vi "zadanie 3.vi"() -> ()   [LabVIEW 2013]
panel:
  out "Meter":dbl(knob) scale=0.0..1.0
  in  "Управление":bool
  out "Напряжение":dbl[](graph)
  out "Тестовый массив":dbl[](array[numeric])
  in  "С":dbl
  out "Заряд стикающий с конденсатора":dbl[](graph)
  out "Сила тока на нагрузке":dbl[](graph)
  out "t":dbl
  out "I":dbl
  out "Q":dbl
  in  "R":dbl
  in  "ЭДС":dbl
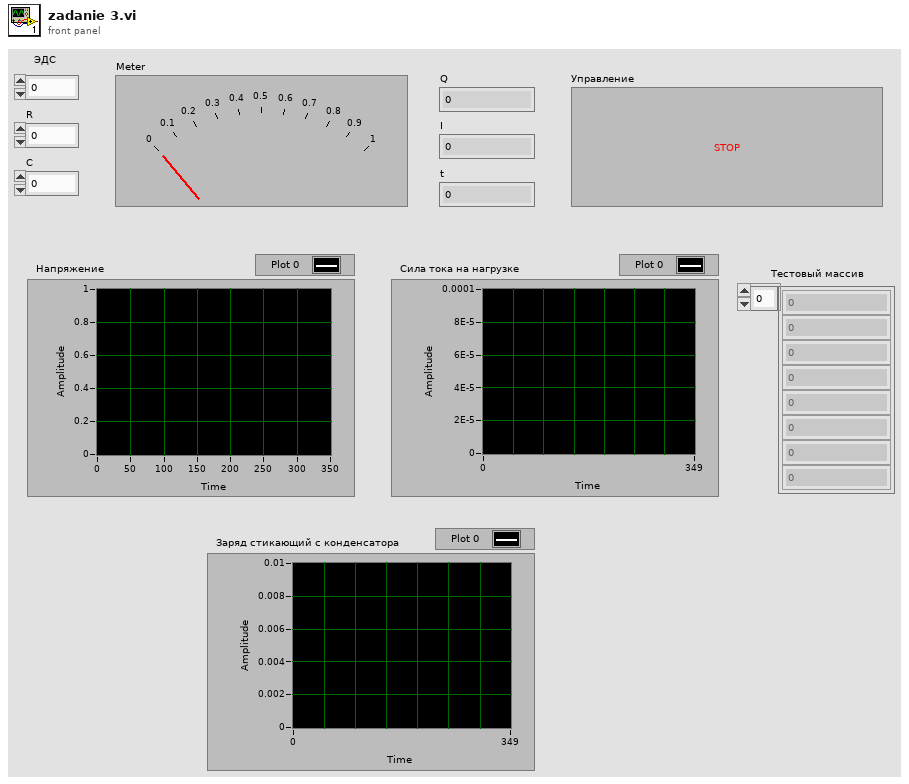
[diagram p1: front panel]
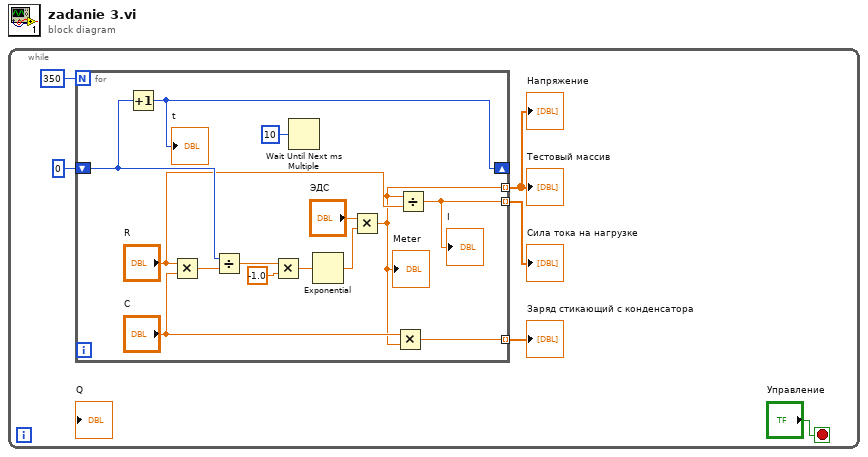
[diagram p0: block diagram]
diagram:
  n1 = while {
    stop <- "Управление" stop-if-true
    n2 = for {
      N: 350 -> [_]
      tunnel: [w8] -> w1 mode=indexing
      shift-right: [w10] -> _
      shift-left: 0 -> [w14]
      tunnel: [w9] -> w4 mode=indexing
      tunnel: [w11] -> w3 mode=indexing
      n3 = Increment(x=w14) -> (x+1=w10:i32)
      "t" <- w10
      n4 = Multiply(x="R", y="С") -> (x*y=w20:dbl)
      n5 = Divide(x=w14, y=w20) -> (x/y=w19:dbl)
      n6 = Multiply(x=w19, y=-1.0) -> (x*y=w15:dbl)
      n7 = Wait Until Next ms Multiple(millisecond multiple=u32 10) -> ()  [unwired: 1 out]
      n8 = Exponential(1:w15) -> (0:w16:dbl)
      n9 = Multiply(x="ЭДС", y=w16) -> (x*y=w8:dbl)
      "Meter" <- w8
      n10 = Multiply(x="С", y=w8) -> (x*y=w11:dbl)
      n11 = Divide(x=w8, y="R") -> (x/y=w9:dbl)
      "I" <- w9
    }
    "Сила тока на нагрузке" <- w4
    "Заряд стикающий с конденсатора" <- w3
    "Тестовый массив" <- w1
    "Напряжение" <- w1
  }
